vi "SAMPLE_lv_icon.vi"(10 "Color icon in":T1, 11 "BW icon in":T1) -> (0 "Error code out":i32, 2 "Color icon out":T1, 3 "BW icon out":T1)   [LabVIEW 2021, in "lv_icon.lvlib"]
uses:
  <vilib>/picture/picture.llb/imagedata.ctl
  <vilib>/LabVIEW Icon API/lv_icon/lv_icon.lvlib
panel:
  out "The icon will be set to this:":picture
  in  "OK Button":bool
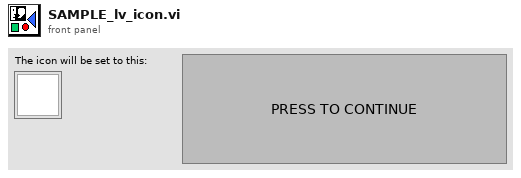
[diagram p1: front panel]
types:
  T1 = typedef "imagedata.ctl" = cluster{"image type":i32, "image depth":i32, "image":u8[], "mask":u8[], "colors":u32[], "Rectangle":cluster{"left":i16, "top":i16, "right":i16, "bottom":i16}}
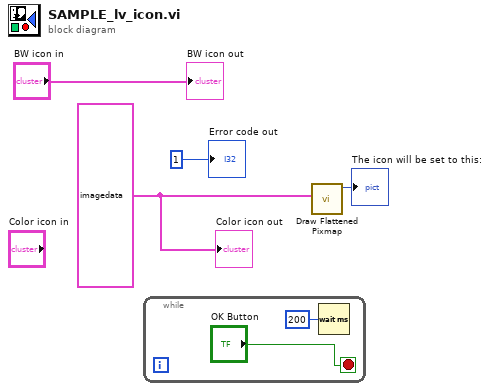
[diagram p0: block diagram]
diagram:
  w2 = T1 {"image type"=0, "image depth"=24, "image"=array[3072 elements], "mask"=[], "colors"=[], "Rectangle"={"left"=0, "top"=0, "right"=32, "bottom"=32}} ("image data")
  n1 = while {
    stop <- "OK Button" stop-if-true
    n2 = Wait (ms)(milliseconds to wait=u32 200) -> ()  [unwired: 1 out]
  }
  n3 = call <vilib>:"Draw Flattened Pixmap.vi"("image data"=w2) -> ("new picture"=→"The icon will be set to this:":picture)  [unwired: 8 in]
  "BW icon out" <- "BW icon in"
  "Color icon out" <- w2
  "Error code out" <- 1 ("code")
